vi "Table_Add Test Result.vi"(7 "Pass?":bool, 8 "error in (no error)":errorcluster, 9 "Test Result":string, 10 "index (row)":i32=5, 11 "Table in":refnum<vi>) -> (0 "error out":errorcluster)   [LabVIEW 2025]
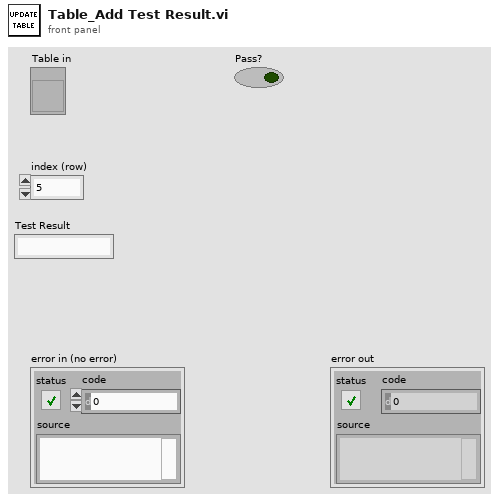
[diagram p1: front panel]
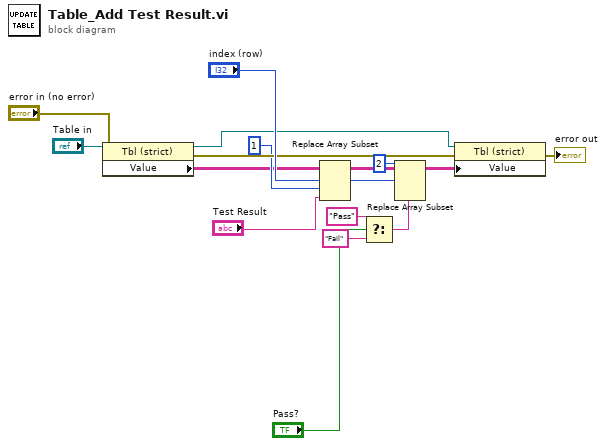
[diagram p0: block diagram]
diagram:
  n1 = property class="Tbl (strict)"(reference="Table in", error in="error in (no error)") -> (reference out=w13:refnum<vi>, error out=w12:errorcluster, "Value"=w3:string[][])
  n2 = Replace Array Subset(array=w3, new element="Test Result", index (row)="index (row)", index (col)=1 ("disabled index (col)")) -> (w5:string[][])
  n3 = Select(t="Pass", s="Pass?", f="Fail") -> (s? t:f=w6:string)
  n4 = Replace Array Subset(array=w5, new element=w6, index (row)="index (row)", index (col)=2 ("disabled index (col)")) -> (w11:string[][])
  n5 = property class="Tbl (strict)"(reference=w13, error in=w12, "Value"=w11) -> (error out=→"error out":errorcluster)  [unwired: 1 out]
